vi "Close Device.vi"(8 "error in (no error)":errorcluster, 10 "Handle":u32, 11 "ThAr in":refnum<class "ThAr.lvclass">) -> (0 "error out":errorcluster, 3 "ThAr out":refnum<class "ThAr.lvclass">)   [LabVIEW 2016, in "ThAr.lvclass"]
uses:
  ThAr.lvclass
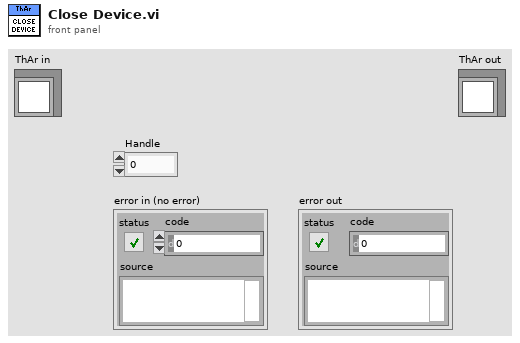
[diagram p1: front panel]
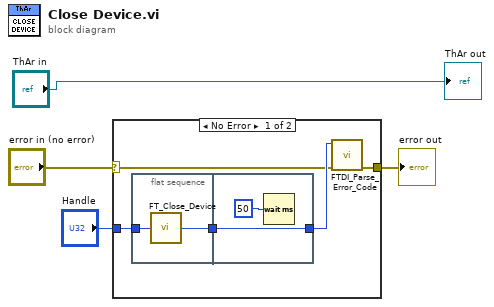
[diagram p0: block diagram]
diagram:
  n1 = case shown="No Error" "error in (no error)" {
    selector: "error in (no error)" -> [w5 w14]
    tunnel: [w9 w14] -> w4
    tunnel: "Handle" -> [w7 _]
    frame No Error {
      n2 = flat-sequence {
        tunnel: w7 -> [w10]
        tunnel: [w11] -> w6
        tunnel: [w13] -> w8
        tunnel: w6 -> [w13]
        frame #0 {
          n3 = call "FT_Close_Device.vi"("Handle"=w10) -> ("FT_Status"=w11:u32)
        }
        frame #1 {
          n4 = Wait (ms)(milliseconds to wait=u32 50) -> ()  [unwired: 1 out]
        }
      }
      n5 = call "FTDI_Parse_Error_Code.vi"("error in (no error)"=w5, "FT_Status"=w8) -> ("error out"=w9:errorcluster)  [unwired: 9 in]
    }
    frame Error {
    }
  }
  "error out" <- w4
  "ThAr out" <- "ThAr in"
